vi "fftw__free_poly.vi"   [LabVIEW 2020, in "FFTWDLL.lvlib"]
doc: "Free FFTW memory block."
uses:
  FFTWDLL.lvlib
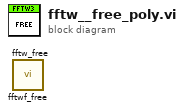
[diagram p0: block diagram]
diagram:
  n1 = call "fftwf_free.vi"() -> ()  [unwired: 11 in, 1 out]
  n2 = call "fftw_free.vi"() -> ()  [unwired: 11 in, 1 out]
